vi "INIstringToVariant.vi"(5 "type":variant=variant(dbl[] []), 7 "use system decimal point (T)":bool=TRUE, 10 "Section Name (empty: type label)":string, 11 "INI Content":string) -> (2 "Value Class":T1, 3 "Variant-formatted Value":variant)   [LabVIEW 2013, in "OpenSerializer.lvlib" / "Serializer.PlainText.INI.lvclass"]
uses:
  Serializer.PlainText.INI.lvclass
  Serializer.PlainText/Character Class -- Enum.ctl
  <vilib>/LabVIEW Open Source Project/Data Manipulation/TypeDescriptor/TypeDescriptor_GetName.vi
  <vilib>/LabVIEW Open Source Project/Data Manipulation/TypeDescriptor/TypeDescriptor_GetPString.vi
  Serializer.PlainText/Serializer.PlainText.lvclass
  <vilib>/LabVIEW Open Source Project/Data Manipulation/Variant/OpenVariant.lvlib
  <vilib>/Utility/VariantDataType/VariantType.lvlib
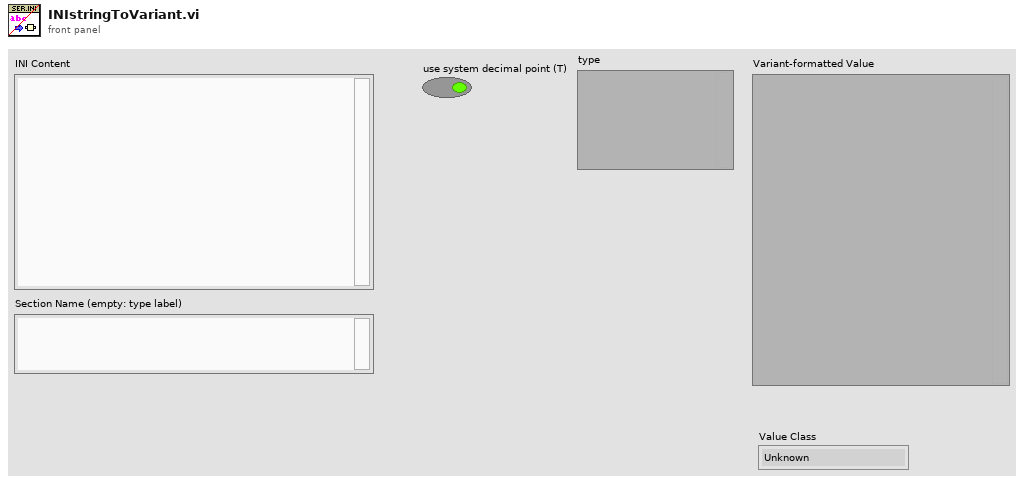
[diagram p1: front panel]
types:
  T1 = typedef "OpenSerializer.lvlib/Serializer.PlainText.lvclass/Character Class -- Enum.ctl" = enum16{"Unknown", "Sign", "Zero", "Integer", "Float", "Complex", "Scientific", "Engineering", "Hexadecimal", "Binary", "Decimal", "Octal", "Unit", "Invalid", "Timestamp", "Boolean", "String", "Path", "null", "cluster", "array"}
  T2 = typedef "VariantType.lvlib/Type.ctl" = enum8{"Invalid Type", "Void", "I8", "I16", "I32", "I64", "U8", "U16", "U32", "U64", "Single Float", "Double Float", "Extended Float", "Single Complex", "Double Complex", "Extended Complex", "Enum U8", "Enum U16", "Enum U32", "Enum U64", "Single Float With Unit", "Double Float With Unit", "Extended Float With Unit", "Single Complex with Unit", "Double Complex with Unit", "Extended Complex with Unit", "Boolean", "String", "Path", "Picture", "Tag", "Array", "Cluster", "Variant", "LV Variant", "Waveform", "Timestamp", "Digital Waveform", "Digital Data", "ExpressData", "Refnum", "External Data", "VI", "Poly VI", "LabVIEW Class Instance", "Fixed Point"}
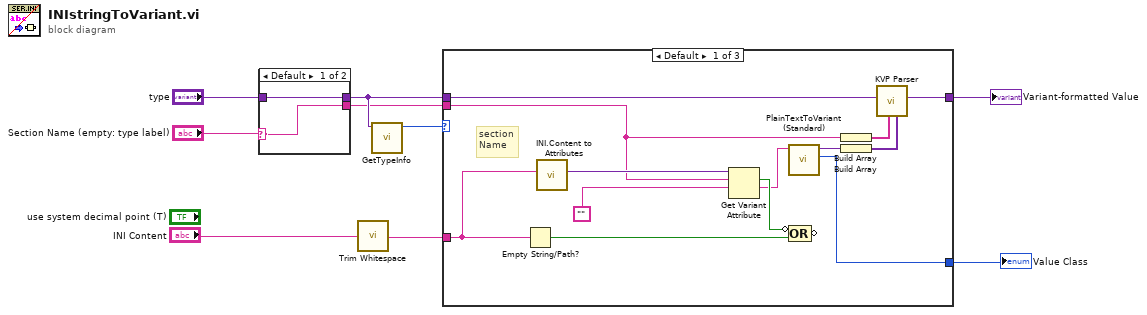
[diagram p0: block diagram]
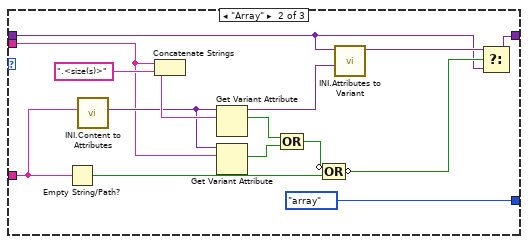
[diagram p2: hidden frame]
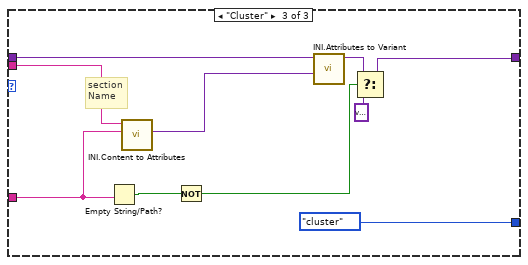
[diagram p3: hidden frame]
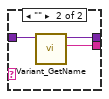
[diagram p4: hidden frame]
diagram:
  n1 = case shown="Default" "Section Name (empty: type label)" {
    selector: "Section Name (empty: type label)" -> [w10 _]
    tunnel: "type" -> [w11 w14]
    tunnel: [w11 w13] -> w2
    tunnel: [w10 w12] -> w1
    frame Default {
    }
    frame "" {
      n2 = call <vilib>:"Variant_GetName.vi"("Variant"=w14) -> ("Name"=w12:string, "Variant dup"=w13:variant)  [unwired: 8 in, 1 out]
    }
  }
  n3 = call <vilib>:"Trim Whitespace.vi"("string"="INI Content") -> ("trimmed string"=w4:string)  [unwired: 1 in]
  n4 = call <vilib>:"GetTypeInfo.vi"("Variant"=w2) -> ("Type Enum"=w3:T2)  [unwired: 6 in, 4 out]
  n5 = case shown="Default" w3 {
    tunnel: w2 -> [w22 w28 w44]
    tunnel: w4 -> [w25 w39 w51]
    tunnel: [w15 Character_Class_--_Enum."array" ("Value Class") Character_Class_--_Enum."cluster" ("Value Class")] -> w7
    tunnel: w1 -> [w20 w33 w49]
    tunnel: [w18 w35 w43] -> w8
    frame Default {
      # "section\nName"
      n6 = Empty String/Path?(string/path=w25) -> (empty?=w27:bool)
      n7 = call "INI.Content to Attributes.vi"("Content"=w25) -> ("Section Attributes"=w24:variant)  [unwired: 10 in]
      n8 = Get Variant Attribute(Variant=w24, name=w20, default value (empty Variant)="") -> (found=w26:bool, value=w17:string)  [unwired: 1 in, 2 out]
      n9 = call "PlainTextToVariant (Standard).vi"("String-formatted Value"=w17) -> ("Value Class"=w15:T1, "Variant-formatted Value"=w16:variant)  [unwired: 9 in]
      n10 = Compound Arithmetic op=OR(invert w26, w27) -> ()  [unwired: 1 out]
      n11 = Build Array(w20) -> (w21:string[])
      n12 = Build Array(w16) -> (w23:variant[])
      n13 = call <vilib>:"KVP Parser.vi"("Values"=w23, "Keys"=w21, "Default Value"=w22) -> ("Value"=w18:variant)  [unwired: 5 in, 3 out]
    }
    frame "Array" {
      n14 = Empty String/Path?(string/path=w39) -> (empty?=w42:bool)
      n15 = call "INI.Content to Attributes.vi"("Content"=w39) -> ("Section Attributes"=w34:variant)  [unwired: 10 in]
      n16 = Concatenate Strings(w33, ".<size(s)>" ("string")) -> (w41:string)
      n17 = Get Variant Attribute(Variant=w34, name=w41) -> (duplicate Variant=w37:variant, found=w31:bool)  [unwired: 2 in, 2 out]
      n18 = Get Variant Attribute(Variant=w34, name=w33) -> (found=w32:bool)  [unwired: 2 in, 3 out]
      n19 = Compound Arithmetic op=OR(w31, w32) -> (w30:bool)
      n20 = Compound Arithmetic op=OR(invert w30, w42) -> (invert w36:bool)
      n21 = call "INI.Attributes to Variant.vi"("Section Attribute"=w37, "Datatype"=w28) -> ("Variant"=w29:variant)  [unwired: 8 in, 1 out]
      n22 = Select(t=w29, s=w36, f=w28) -> (s? t:f=w35:variant)
    }
    frame "Cluster" {
      # "section\nName"
      n23 = Empty String/Path?(string/path=w51) -> (empty?=w52:bool)
      n24 = call "INI.Content to Attributes.vi"("Content"=w51, "Section Name"=w49) -> ("Section Attributes"=w48:variant)  [unwired: 9 in]
      n25 = Not(x=w52) -> (.not. x?=w45:bool)
      n26 = call "INI.Attributes to Variant.vi"("Section Attribute"=w48, "Datatype"=w44) -> ("Variant"=w46:variant)  [unwired: 8 in, 1 out]
      n27 = Select(t=w46, s=w45, f=variant ("y")) -> (s? t:f=w43:variant)
    }
  }
  "Variant-formatted Value" <- w8
  "Value Class" <- w7
